vi "Recursive Search for Protected VIs.vi"(8 "error in (no error)":errorcluster, 9 "Scope":T1(ring)=enum."protected", 10 "Recursive Referemce":refnum<vi>, 11 "LVClassLibrary in":refnum<vi>) -> (0 "error out":errorcluster, 2 "Protected VI Refs":refnum<vi>[](array[refnum]), 3 "LVClassLibrary out":refnum<vi>)   [LabVIEW 2020, in "Test Double Factory.lvclass"]
uses:
  Test Double Factory.lvclass
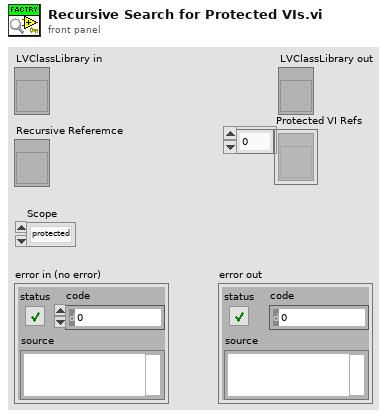
[diagram p1: front panel]
types:
  T1 = enum32{"invalid scope", "public", "private", "protected", "community"}
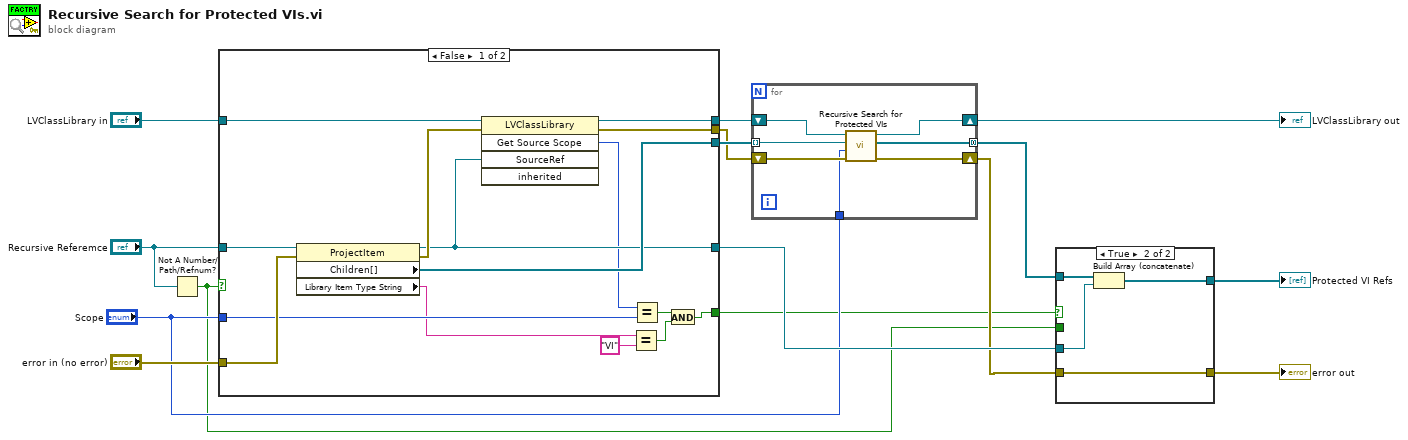
[diagram p0: block diagram]
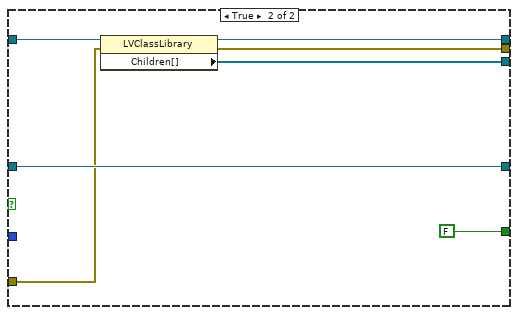
[diagram p2: hidden frame]
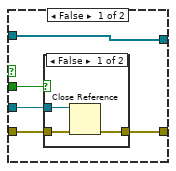
[diagram p3: hidden frame]
diagram:
  n1 = Not A Number/Path/Refnum?(number/path/refnum="Recursive Referemce") -> (NaN/Path/Refnum?=w1:bool)
  n2 = case shown="False" w1 {
    tunnel: "LVClassLibrary in" -> [w26 w37]
    tunnel: [w27 w36] -> w14
    tunnel: [w23 w35] -> w10
    tunnel: [w30 w34] -> w9
    tunnel: "Recursive Referemce" -> [w29 w35]
    tunnel: "error in (no error)" -> [w28 w32]
    tunnel: [w24 w33] -> w6
    tunnel: "Scope" -> [w22 _]
    tunnel: [w19 FALSE] -> w2
    frame False {
      n3 = property class="ProjectItem"(reference=w29, error in=w28) -> (reference out=w23:refnum<vi>, error out=w25:errorcluster, "Children[]"=w30:refnum<vi>[], "Library Item Type String"=w17:string)
      n4 = invoke class="LVClassLibrary" method="Get Source Scope"(reference=w26, error in=w25, "SourceRef"=w23) -> (reference out=w27:refnum<vi>, error out=w24:errorcluster, "GetSourceScope"=w21:T1)  [unwired: 2 in, 2 out]
      n5 = Equal?(x=w17, y="VI") -> (x = y?=w18:bool)
      n6 = Equal?(x=w21, y=w22) -> (x = y?=w20:bool)
      n7 = And(x=w20, y=w18) -> (x .and. y?=w19:bool)
    }
    frame True {
      n8 = property class="LVClassLibrary"(reference=w37, error in=w32) -> (reference out=w36:refnum<vi>, error out=w33:errorcluster, "Children[]"=w34:refnum<vi>[])
    }
  }
  n9 = for {
    tunnel: w9 -> [w44] mode=indexing
    shift-right: [w42] -> w13
    shift-left: w14 -> [w43]
    tunnel: [w41] -> w11 mode=concatenating
    shift-right: [w39] -> w5
    shift-left: w6 -> [w40]
    tunnel: "Scope" -> [w38]
    n10 = call "Recursive Search for Protected VIs.vi"("error in (no error)"=w40, "Scope"=w38, "Recursive Referemce"=w44, "LVClassLibrary in"=w43) -> ("error out"=w39:errorcluster, "Protected VI Refs"=w41:refnum<vi>[], "LVClassLibrary out"=w42:refnum<vi>)  [unwired: 5 in]
  }
  "LVClassLibrary out" <- w13
  n11 = case shown="True" w2 {
    tunnel: w10 -> [w46 w57]
    tunnel: [w49 w56] -> w12
    tunnel: w11 -> [w49 w55]
    tunnel: w5 -> [w48 w54]
    tunnel: [w47 w54] -> w4
    tunnel: w1 -> [w45 _]
    frame False {
      n12 = case shown="False" w45 {
        tunnel: w48 -> [w52 w53]
        tunnel: [w51 w53] -> w47
        tunnel: w46 -> [w50 _]
        frame False {
          n13 = Close Reference(reference=w50, error in (no error)=w52) -> (error out=w51:errorcluster)
        }
        frame True {
        }
      }
    }
    frame True {
      n14 = Build Array (concatenate)(w55, w57) -> (w56:refnum<vi>[])
    }
  }
  "error out" <- w4
  "Protected VI Refs" <- w12
